vi "Reshape to ROI.vi"(10 "PicamRoi":T1, 11 "Array in":u16[](array[numeric])) -> (3 "Array out 2":u16[][](array[numeric]))   [LabVIEW 2019, in "Picam.lvclass"]
uses:
  Picam.lvclass
  picam32_LabView_SDK/PICam_lib/types/PicamRoi.ctl
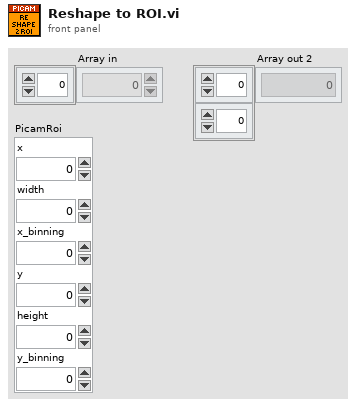
[diagram p1: front panel]
types:
  T1 = typedef "PicamRoi.ctl" = cluster{"x":i32, "width":i32, "x_binning":i32, "y":i32, "height":i32, "y_binning":i32}
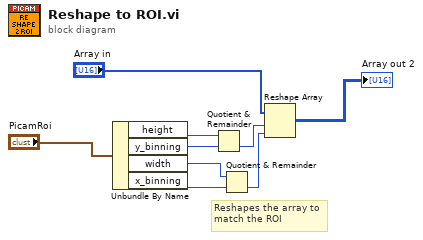
[diagram p0: block diagram]
diagram:
  # "Reshapes the array to\nmatch the ROI"
  n1 = Unbundle By Name("PicamRoi") -> ("height"=w3:i32, "y_binning"=w4:i32, "width"=w6:i32, "x_binning"=w7:i32)
  n2 = Quotient & Remainder(x=w3, y=w4) -> (floor(x/y)=w5:i32)  [unwired: 1 out]
  n3 = Quotient & Remainder(x=w6, y=w7) -> (floor(x/y)=w8:i32)  [unwired: 1 out]
  n4 = Reshape Array("Array in", w5, w8) -> (→"Array out 2":u16[][])
